vi "Gas Scheduler.vi"(0 "Path to Program File":path) -> (2 "Microbalance\nN2":dbl, 3 "N2":dbl, 4 "H2":dbl, 6 "N2 (Wet)":dbl, 7 "Stage":dbl, 8 "CO2":dbl, 9 "Stage Time":dbl, 10 "Flow 7":dbl, 11 "Elapsed Time":dbl, 14 "O2":dbl, 15 "Flow 8":dbl)   [LabVIEW 2018]
uses:
  <vilib>/MakerHub/LINX/Public/Utilities/Open Serial.vi
  <vilib>/MakerHub/LINX/Public/Sensors/Motion/Servo/Servo Open One Channel.vi
  <vilib>/MakerHub/LINX/Public/Sensors/Motion/Servo/Servo Set Pulse Width One Channel.vi
  Instance           1 42Saved   8 Ch Gas Scheduler with Controller .vi
  <vilib>/Utility/file.llb/Write Delimited Spreadsheet (DBL).vi
  <vilib>/Utility/file.llb/Read Delimited Spreadsheet (DBL).vi
  <vilib>/MakerHub/LINX/Public/Sensors/Motion/Servo/Servo Close One Channel.vi
  <vilib>/MakerHub/LINX/Public/Sensors/Motion/Servo/Servo.lvlib
  <vilib>/MakerHub/LINX/LMH-LINX.lvlib
panel:
  in  "Recording Peroid":dbl
  in  "Comments":string
  out "Act Flow 8":dbl
  out "Act Flow 7":dbl
  out "Act Flow 6":dbl
  out "Act Flow 5":dbl
  out "Act Flow 4":dbl
  out "Act Flow 3":dbl
  out "Act Flow 2":dbl
  out "Act Flow 1":dbl
  in  "Start Gas Program":bool
  in  "Servo Channel":u8=11
  in  "Arduino Port":refnum<visa-resource-name>="COM7"
  in  "?":bool
  in  "MFC Com Port":refnum<visa-resource-name>="COM5"
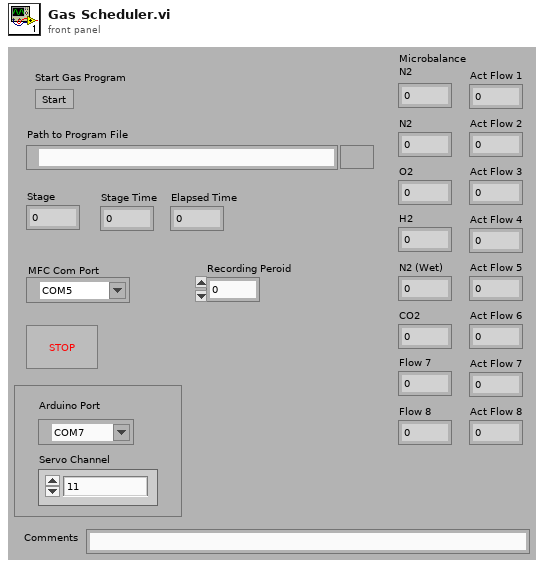
[diagram p1: front panel]
types:
  T1 = typedef "LMH-LINX.lvlib/LINX Ref.ctl" = cluster{"IO":T2, "Interface":T3, "LINX Device Config":T4}
  T2 = typedef "LMH-LINX.lvlib/Platform.ctl" = enum16{"Remote", "Local"}
  T3 = typedef "LMH-LINX.lvlib/Interface.ctl" = enum16{"Serial", "TCP"}
  T4 = typedef "LMH-LINX.lvlib/Device.lvlib/LINX Device Config.ctl" = cluster{"Interface":T3, "COM Port":refnum<visa-resource-name>, "TCP Configuration":T5, "Device Family":u8, "Device ID":u8, "Device Name":string, "TCP Ref":refnum<k5>, "Channels":T6}
  T5 = typedef "LMH-LINX.lvlib/Device.lvlib/TCP Config.ctl" = cluster{"IP Address":string, "Port":u16}
  T6 = typedef "LMH-LINX.lvlib/Channels.ctl" = cluster{"DI":u8[], "DO":u8[], "AI":u8[], "AO":u8[], "PWM":u8[], "QE":u8[], "UART":u8[], "I2C 2":u8[], "SPI":u8[], "CAN":u8[], "Servo":u8[], "AI Ref (V)":dbl, "AI Resolution (Bits)":u8, "AO Ref (V)":dbl, "AO Resolution (Bits)":u8}
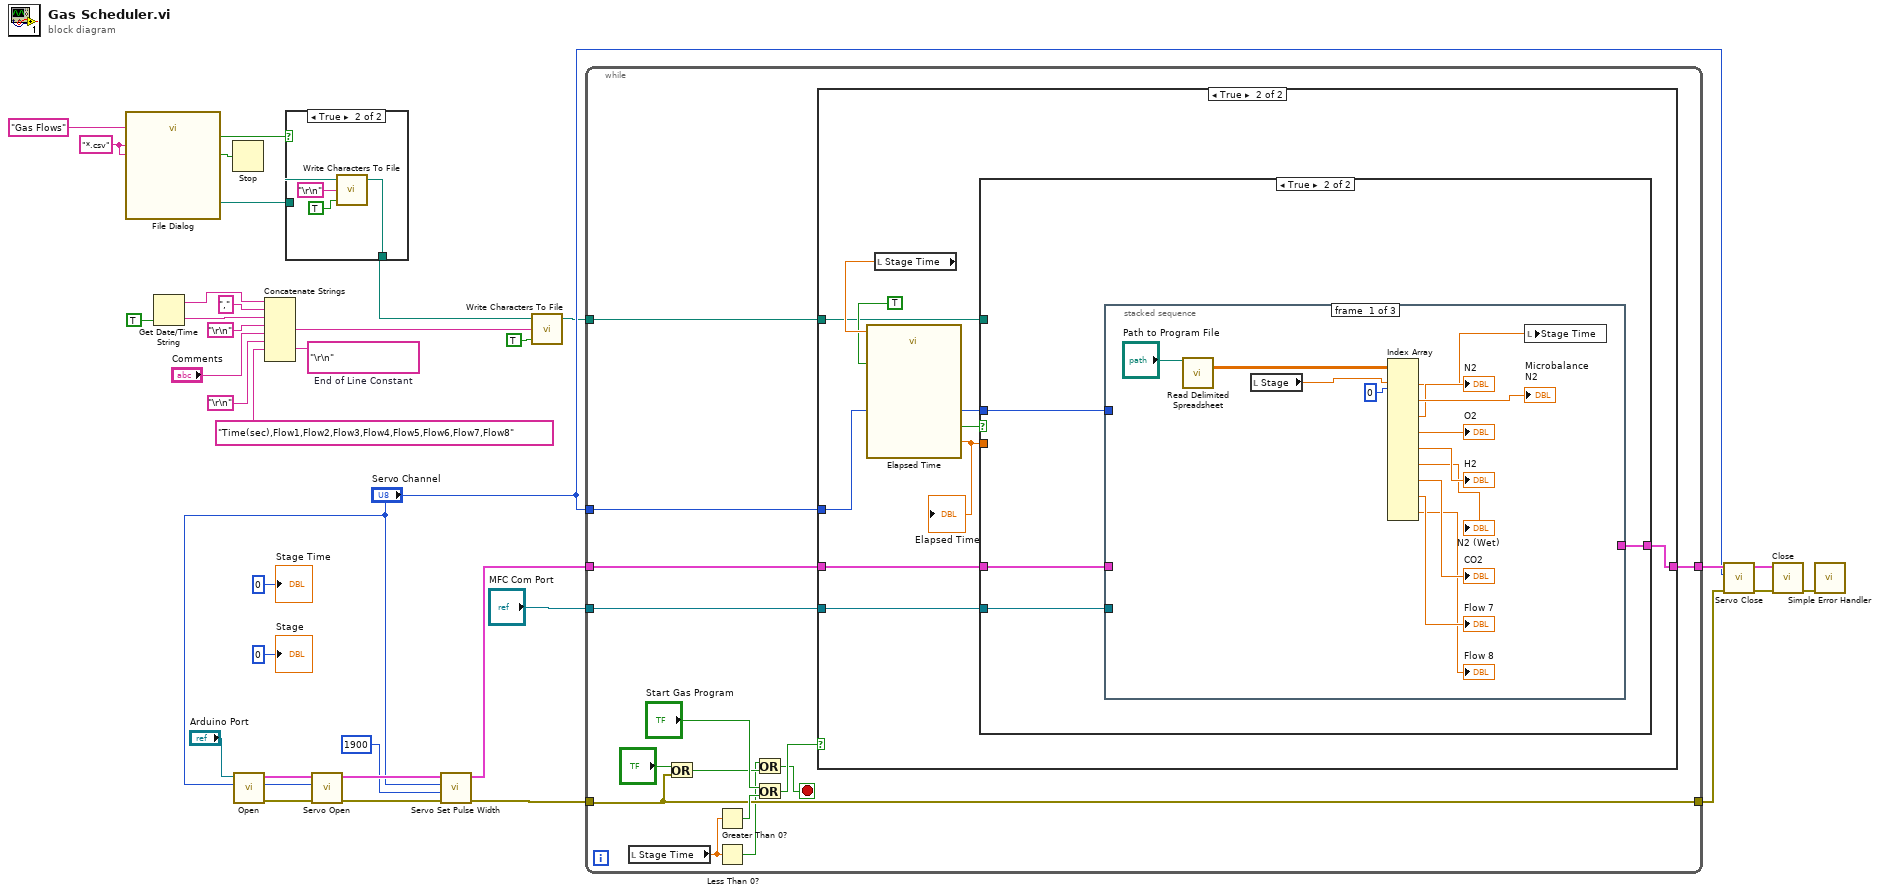
[diagram p0: block diagram]
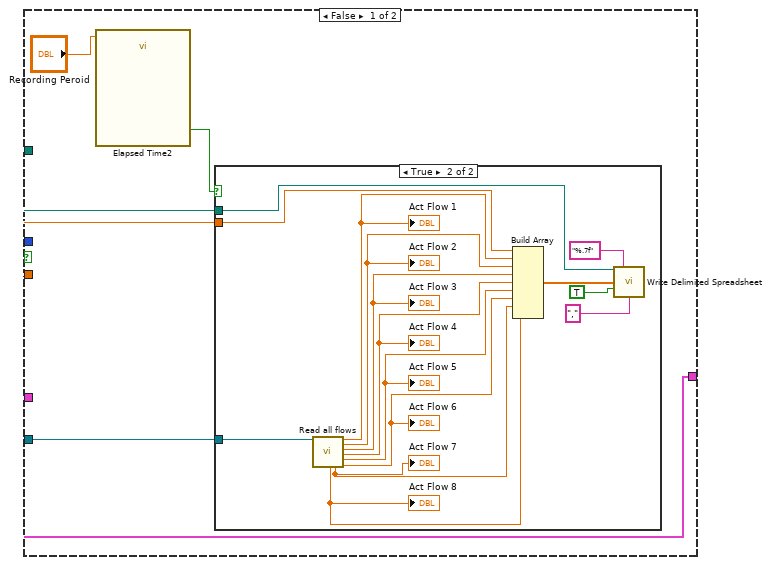
[diagram p4: hidden frame]
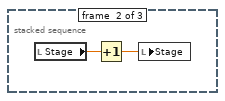
[diagram p6: hidden frame]
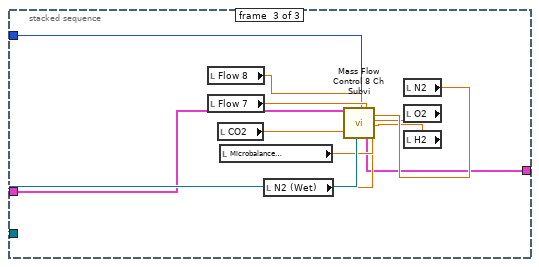
[diagram p7: hidden frame]
diagram:
  w8 = "*.csv"
  w14 = "\r\n"  # End of Line Constant
  n1 = call "File Dialog"("default name"="Gas Flows", "pattern (all files)"=w8, "pattern label"=w8) -> ("selected path"=w2:path, "exists"=w3:bool, "cancelled"=w6:bool)  [unwired: 9 in, 1 out]
  n2 = Get Date/Time String(want seconds? (F)=TRUE) -> (date string=w5:string, time string=w13:string)  [unwired: 2 in]
  n3 = Stop(stop? (T)=w6) -> ()
  n4 = call-poly <vilib>:"Open.vi"("Serial Port"="Arduino Port") -> ("Error Out"=w25:errorcluster, "LINX Resource"=w27:T1)  [unwired: 8 in, 1 out]
  n5 = Concatenate Strings "Concatenate Strings"(w5, ",", w13, "\r\n", "Comments", "\r\n", "Time(sec),Flow1,Flow2,Flow3,Flow4,Flow5,Flow6,Flow7,Flow8" ("string"), w14) -> (w18:string)
  n6 = case shown="True" w3 {
    tunnel: w2 -> [w36 w38]
    tunnel: [w36 w37] -> w1
    frame False {
    }
    frame True {
      n7 = call <vilib>:"Write Characters To File.vi"("append to file? (new file:F)"=TRUE, "character string"="\r\n", "file path (dialog if empty)"=w38) -> ("new file path (Not A Path if cancelled)"=w37:path)  [unwired: 2 in]
    }
  }
  n8 = call-poly <vilib>:"Servo Open.vi"("Error In"=w25, "Servo Channel"="Servo Channel", "LINX Resource"=w27) -> ("Error Out"=w21:errorcluster, "LINX Resource"=w24:T1)  [unwired: 7 in]
  n9 = call-poly <vilib>:"Servo Set Pulse Width.vi"("Error In"=w21, "Pulse Width (uS)"=1900, "Servo Channel"="Servo Channel", "LINX Resource"=w24) -> ("Error Out"=w22:errorcluster, "LINX Resource"=w23:T1)  [unwired: 6 in]
  n10 = call <vilib>:"Write Characters To File.vi"("append to file? (new file:F)"=TRUE, "character string"=w18, "file path (dialog if empty)"=w1) -> ("new file path (Not A Path if cancelled)"=w9:path)  [unwired: 2 in]
  n11 = while {
    tunnel: "MFC Com Port" -> [w52]
    tunnel: "Servo Channel" -> [w49]
    tunnel: [w51] -> w29
    tunnel: [w47] -> w28
    tunnel: w23 -> [w48]
    tunnel: w22 -> [w47]
    tunnel: w9 -> [w41]
    stop <- w42 stop-if-true
    n12 = local read "Stage Time"() -> (w45:dbl)
    n13 = Or(x="?", y=w47) -> (x .or. y?=w44:bool)
    n14 = Greater Than 0?(x=w45) -> (x > 0?=w53:bool)
    n15 = Less Than 0?(x=w45) -> (x < 0?=w43:bool)
    n16 = Or(x=w43, y=w44) -> (x .or. y?=w42:bool)
    n17 = Or(x="Start Gas Program", y=w53) -> (x .or. y?=w54:bool)
    n18 = case shown="True" w54 {
      tunnel: w52 -> [_ w61]
      tunnel: w48 -> [w55 w59]
      tunnel: [w55 w60] -> w51
      tunnel: w49 -> [_ w58]
      tunnel: w41 -> [_ w57]
      frame False {
      }
      frame True {
        n19 = local read "Stage Time"() -> (w64:dbl)
        n20 = call "Elapsed Time"("Time Target (s)"=w64, "Auto Reset"=TRUE) -> ("Elapsed Time (s)"=w56:dbl, "Time has Elapsed"=w62:bool)  [unwired: 10 in, 6 out]
        "Elapsed Time" <- w56
        n21 = case shown="True" w62 {
          tunnel: w61 -> [w69 w89]
          tunnel: w59 -> [w70 w88]
          tunnel: [w70 w87] -> w60
          tunnel: w58 -> [_ w86]
          tunnel: w57 -> [w68 _]
          tunnel: w56 -> [w67 _]
          frame False {
            n22 = call "Elapsed Time2"("Time Target (s)"="Recording Peroid") -> ("Time has Elapsed"=w66:bool)  [unwired: 11 in, 7 out]
            n23 = case shown="True" w66 {
              tunnel: w69 -> [_ w85]
              tunnel: w68 -> [_ w81]
              tunnel: w67 -> [_ w72]
              frame False {
              }
              frame True {
                n24 = call <instrlib>:"Read all flows.vi"("VISA resource name"=w85) -> ("Flow 8"=w80:dbl, "Flow 7"=w79:dbl, "Flow 1"=w73:dbl, "Flow 2"=w74:dbl, "Flow 3"=w75:dbl, "Flow 4"=w76:dbl, "Flow 5"=w77:dbl, "Flow 6"=w78:dbl)  [unwired: 11 in]
                "Act Flow 1" <- w73
                "Act Flow 2" <- w74
                "Act Flow 3" <- w75
                "Act Flow 4" <- w76
                "Act Flow 5" <- w77
                "Act Flow 6" <- w78
                "Act Flow 7" <- w79
                "Act Flow 8" <- w80
                n25 = Build Array(w72, w73, w74, w75, w76, w77, w78, w79, w80) -> (w82:dbl[])
                n26 = call-poly <vilib>:"Write Delimited Spreadsheet.vi"("file path (dialog if empty)"=w81, "format (%.3f)"="%.7f", "1D data"=w82, "append to file? (new file:F)"=TRUE, "delimiter (\\t)"=",") -> ()  [unwired: 9 in, 2 out]
              }
            }
          }
          frame True {
            n27 = stacked-sequence {
              tunnel: w89 -> [_ _ w116]
              tunnel: w88 -> [_ _ w106]
              tunnel: [_ _ w107] -> w87
              tunnel: w86 -> [_ _ w105]
              frame #0 {
                n28 = call-poly <vilib>:"Read Delimited Spreadsheet.vi"("file path (dialog if empty)"="Path to Program File") -> ("all rows"=w101:dbl[][])  [unwired: 9 in, 5 out]
                n29 = local read "Stage"() -> (w90:dbl)
                n30 = Index Array(array=w101, index (row) #1=w90, index (col) #1=0) -> (element #1=w91:dbl, element #2=→"Microbalance\nN2":dbl, element #3=→"N2":dbl, element #4=→"O2":dbl, element #5=→"H2":dbl, element #6=→"N2 (Wet)":dbl, element #7=→"CO2":dbl, element #8=→"Flow 7":dbl, element #9=→"Flow 8":dbl)  [unwired: 16 in]
                n31 = local write "Stage Time"(w91) -> ()
              }
              frame #1 {
                n32 = local read "Stage"() -> (w104:dbl)
                n33 = Increment(x=w104) -> (x+1=w103:dbl)
                n34 = local write "Stage"(w103) -> ()
              }
              frame #2 {
                n35 = local read "Flow 8"() -> (w108:dbl)
                n36 = local read "Flow 7"() -> (w109:dbl)
                n37 = local read "CO2"() -> (w110:dbl)
                n38 = local read "Microbalance\nN2"() -> (w115:dbl)
                n39 = local read "N2 (Wet)"() -> (w111:dbl)
                n40 = local read "N2"() -> (w114:dbl)
                n41 = local read "O2"() -> (w113:dbl)
                n42 = local read "H2"() -> (w112:dbl)
                n43 = call <instrlib>:"Mass Flow Control 8 Ch Subvi.vi"("LINX In"=w106, "VISA resource name"=w116, "Servo Channel"=w105, "MFC 8 set point"=w108, "MFC 7 set point"=w109, "MFC 1  set point"=w115, "MFC 2 set point"=w114, "MFC 3 set point"=w113, "MFC 4 set point"=w112, "MFC 5 set point"=w111, "MFC 6 set point"=w110) -> ("LINX Out"=w107:T1)  [unwired: 8 in]
              }
            }
          }
        }
      }
    }
  }
  n44 = call-poly <vilib>:"Servo Close.vi"("Error In"=w28, "Servo Channel"="Servo Channel", "LINX Resource"=w29) -> ("Error Out"=w32:errorcluster, "LINX Resource"=w31:T1)  [unwired: 7 in]
  n45 = call <vilib>:"Close.vi"("Error In"=w32, "LINX Resource"=w31) -> ("Error Out"=w30:errorcluster)  [unwired: 9 in]
  n46 = call <vilib>:"Simple Error Handler.vi"("error in (no error)"=w30) -> ()  [unwired: 4 in, 5 out]
  "Stage" <- 0
  "Stage Time" <- 0
